vi "Right Joystick Button Map (n00b).vi"(1 "Joystick Name":string="Right Joystick") -> (0 "Actions":cluster{"Left-Right":dbl, "Should Fire?":bool})   [LabVIEW 2012]
uses:
  <vilib>/Rock Robotics/WPI/Joystick/WPI_JoystickGetSetRefNum.vi
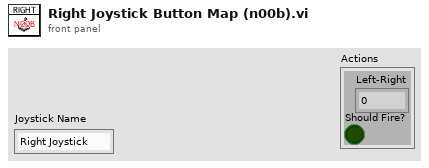
[diagram p1: front panel]
types:
  T1 = typedef "WPI_JoystickDevRef.ctl" = cluster{"Device":T2}
  T2 = typedef "WPI_JoystickDeviceEnum.ctl" = enum16{"USB 1", "USB 2", "USB 3", "USB 4", "Kinect 1", "Kinect 2"}
  T3 = typedef "WPI_JoystickButtonState.ctl" = cluster{"Button 1":bool, "Button 2":bool, "Button 3":bool, "Button 4":bool, "Button 5":bool, "Button 6":bool, "Button 7":bool, "Button 8":bool, "Button 9":bool, "Button 10":bool, "Button 11":bool, "Button 12":bool}
  T4 = cluster{"axis 1 (x)":dbl, "axis 2 (y)":dbl, "axis 3 (throttle)":dbl, "axis 4":dbl, "axis 5":dbl, "axis 6":dbl}
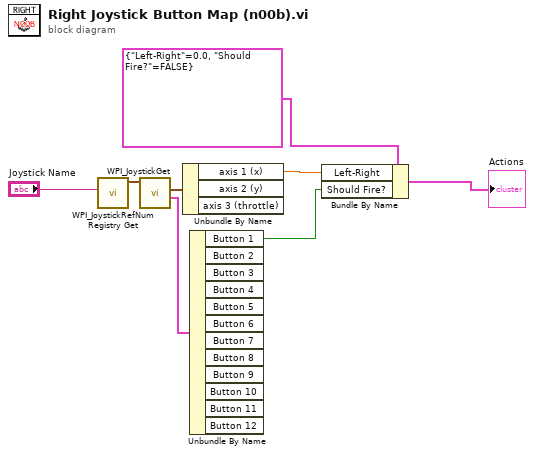
[diagram p0: block diagram]
diagram:
  n1 = call <vilib>:"WPI_JoystickRefNum Registry Get.vi"("refnum name"="Joystick Name") -> ("JoystickDevRef"=w8:T1)  [unwired: 1 in, 9 out]
  n2 = call <vilib>:"WPI_JoystickGet.vi"("JoystickDevRef"=w8) -> ("Buttons"=w5:T3, "Axes"=w6:T4)  [unwired: 1 in, 4 out]
  n3 = Unbundle By Name(w6) -> ("axis 1 (x)"=w3:dbl)  [unwired: 2 out]
  n4 = Unbundle By Name(w5) -> ("Button 1"=w1:bool)  [unwired: 11 out]
  n5 = Bundle By Name(cluster=cluster{"Left-Right":dbl, "Should Fire?":bool} {"Left-Right"=0.0, "Should Fire?"=FALSE}, "Left-Right"=w3, "Should Fire?"=w1) -> (→"Actions":cluster{"Left-Right":dbl, "Should Fire?":bool})
